vi "Query_ResonantFrequency_Sub_VI.vi"(9 "error in (no error)":errorcluster, 11 "connection ID":refnum<k5>) -> (0 "error out":errorcluster, 2 "connection ID_out":refnum<k5>, 3 "Resonant Frequencies":string)   [LabVIEW 2017]
panel:
  out "data out":string
  out "*(type *) &x 3":u8
  out "substring":string
  out "data out 2":string
  out "x+y":i32
  out "array":string[](array[string])
  out "*(type *) &x":u8
  # "OUTPUT"
  # "INPUT"
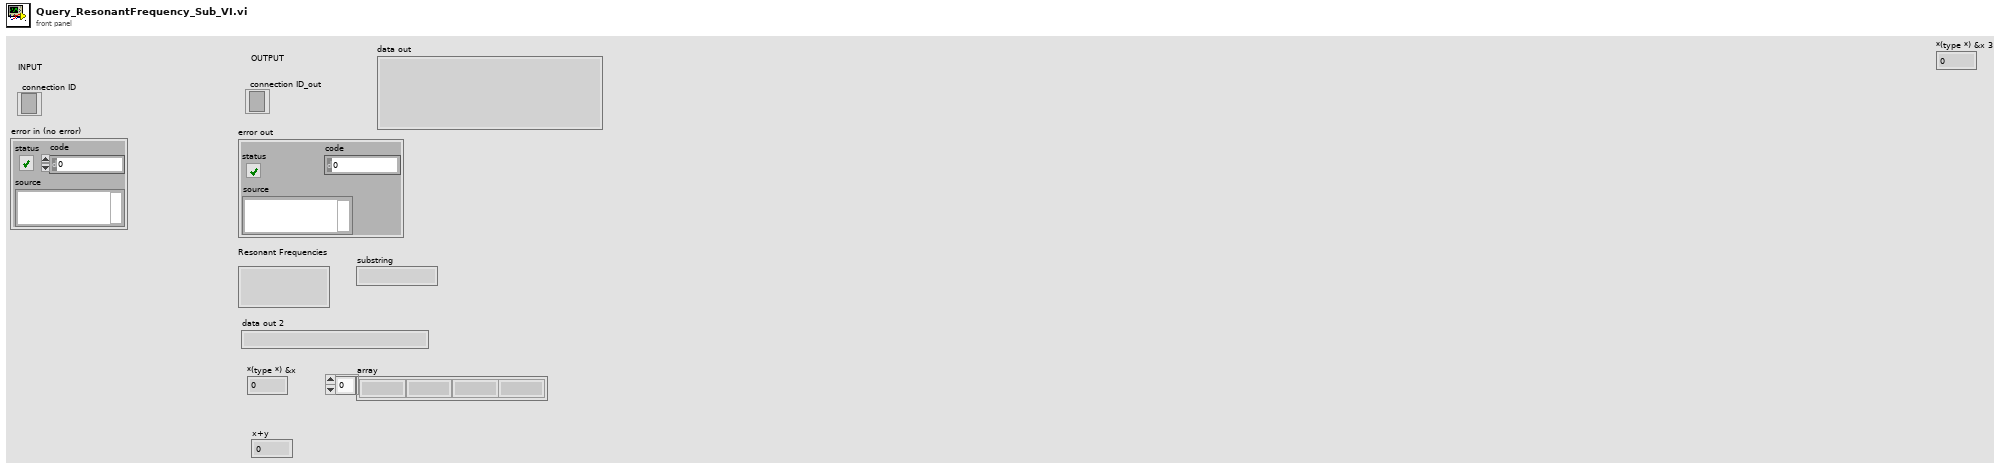
[diagram p1: front panel]
types:
  T1 = enum16{"Standard", "Buffered", "CRLF", "Immediate"}
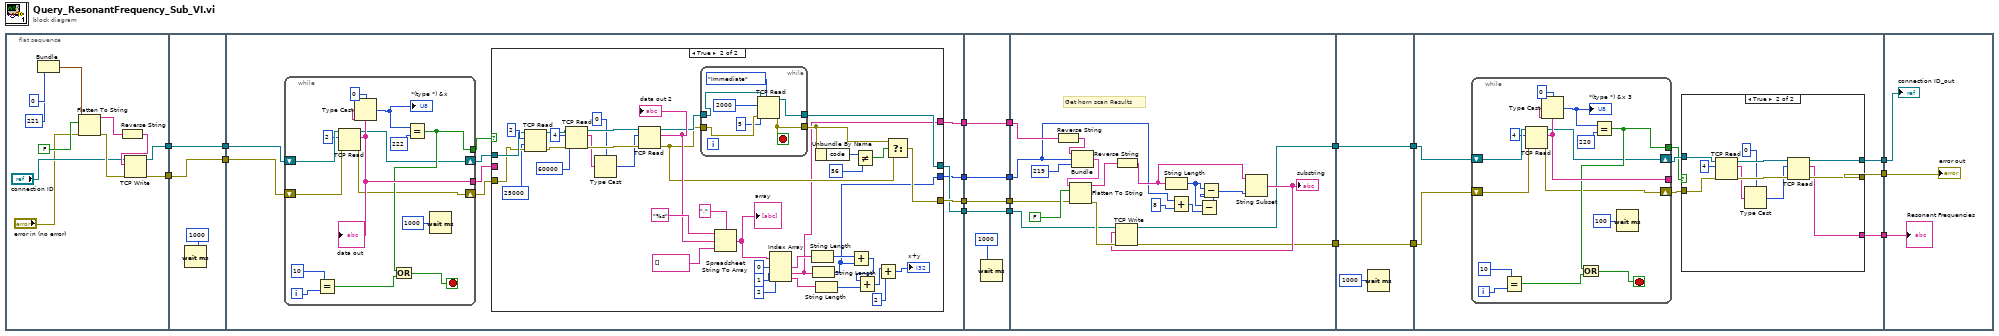
[diagram p0: block diagram]
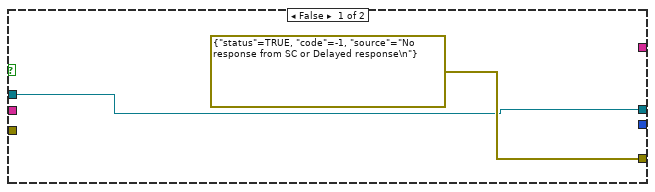
[diagram p2: hidden frame]
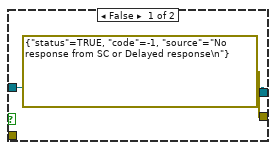
[diagram p3: hidden frame]
diagram:
  n1 = flat-sequence {
    tunnel: [w26] -> w19
    tunnel: [w25] -> w16
    tunnel: w19 -> [w32]
    tunnel: [w32] -> w18
    tunnel: [w31] -> w17
    tunnel: w16 -> [w31]
    tunnel: w18 -> [w41]
    tunnel: w17 -> [w40]
    tunnel: [w38] -> w14
    tunnel: [w36] -> w12
    tunnel: [w35] -> w11
    tunnel: [w34] -> w8
    tunnel: [w110] -> w15
    tunnel: w14 -> [w110]
    tunnel: [w109] -> w13
    tunnel: w12 -> [w109]
    tunnel: w11 -> [w108]
    tunnel: [w108] -> w10
    tunnel: [w107] -> w9
    tunnel: w8 -> [w107]
    tunnel: w15 -> [w127]
    tunnel: w13 -> [w126]
    tunnel: w10 -> [w119]
    tunnel: w9 -> [w124]
    tunnel: [w116] -> w6
    tunnel: [w115] -> w4
    tunnel: [w133] -> w7
    tunnel: w6 -> [w133]
    tunnel: [w132] -> w5
    tunnel: w4 -> [w132]
    tunnel: w7 -> [w141]
    tunnel: w5 -> [w140]
    tunnel: [w138] -> w3
    tunnel: [w137] -> w2
    tunnel: [w136] -> w1
    tunnel: w3 -> [w171]
    tunnel: w2 -> [w170]
    tunnel: w1 -> [w172]
    frame #0 {
      n2 = Bundle(0, 221) -> (w24:cluster{i32, i32})  [unwired: 1 in]
      n3 = Flatten To String(anything=w24, prepend array or string size? (T)=FALSE, error in (no error)="error in (no error)") -> (data string=w23:string, error out=w29:errorcluster)  [unwired: 1 in, 1 out]
      n4 = Reverse String(1:w23) -> (0:w22:string)
      n5 = TCP Write(connection ID="connection ID", data in=w22, error in (no error)=w29) -> (connection ID out=w26:refnum<k5>, error out=w25:errorcluster)  [unwired: 1 in, 1 out]
    }
    frame #1 {
      n6 = Wait (ms)(milliseconds to wait=u32 1000) -> ()  [unwired: 1 out]
    }
    frame #2 {
      n7 = while {
        shift-right: [w47] -> w37
        shift-left: w41 -> [w49]
        shift-right: [w46] -> w39
        shift-left: w40 -> [w48]
        tunnel: [w51] -> w43
        tunnel: [w55] -> w42
        i -> [w54]
        stop <- w52 stop-if-true
        n8 = Equal?(x=10, y=w54) -> (x = y?=w50:bool)
        n9 = TCP Read(connection ID=w49, bytes to read=2, error in (no error)=w48) -> (connection ID out=w47:refnum<k5>, data out=w55:string, error out=w46:errorcluster)  [unwired: 2 in]
        "data out" <- w55
        n10 = Type Cast(type=u8 0, x=w55) -> (*(type *) &x=w57:u8)
        "*(type *) &x" <- w57
        n11 = Equal?(x=w57, y=u8 222) -> (x = y?=w51:bool)
        n12 = Or(x=w51, y=w50) -> (x .or. y?=w52:bool)
        n13 = Wait (ms)(milliseconds to wait=u32 1000) -> ()  [unwired: 1 out]
      }
      n14 = case shown="True" w43 {
        tunnel: w42 -> [_ _]
        tunnel: w39 -> [_ w63]
        tunnel: [errorcluster {"status"=TRUE, "code"=-1, "source"="No response from SC or Delayed response\n"} ("error constant") w69] -> w38
        tunnel: w37 -> [w59 w65]
        tunnel: [w59 w75] -> w36
        tunnel: [_ w67] -> w35
        tunnel: [_ w68] -> w34
        frame False {
        }
        frame True {
          n15 = TCP Read(connection ID=w65, bytes to read=2, error in (no error)=w63, 9:25000 ("timeout ms (25000)")) -> (connection ID out=w64:refnum<k5>, error out=w62:errorcluster)  [unwired: 1 in, 1 out]
          n16 = TCP Read(connection ID=w64, bytes to read=4, error in (no error)=w62, 9:60000 ("timeout ms (25000)")) -> (connection ID out=w82:refnum<k5>, data out=w81:string, error out=w83:errorcluster)  [unwired: 1 in]
          n17 = Type Cast(type=u8 0, x=w81) -> (*(type *) &x=w79:u8)
          n18 = TCP Read(connection ID=w82, bytes to read=w79, error in (no error)=w83) -> (connection ID out=w76:refnum<k5>, data out=w78:string, error out=w70:errorcluster)  [unwired: 2 in]
          "data out 2" <- w78
          n19 = while {
            tunnel: w70 -> [w105]
            tunnel: w76 -> [w106]
            tunnel: [w104] -> w75
            tunnel: [w100] -> w74
            stop <- w100 stop-if-true
            n20 = TCP Read(connection ID=w106, bytes to read=2000, error in (no error)=w105, 7:T1."Immediate" ("mode (standard)"), 9:5 ("timeout ms (25000)")) -> (connection ID out=w104:refnum<k5>, error out=w100:errorcluster)  [unwired: 1 out]
          }
          n21 = Spreadsheet String To Array(delimiter (Tab)=",", format string="%s", spreadsheet string=w78, array type (2D Dbl)=string[] []) -> (array=w96:string[])
          "array" <- w96
          n22 = Index Array(array=w96, index #1=0 ("index"), index #2=1 ("index"), index #3=2 ("index")) -> (element #1=w85:string, element #2=w68:string, element #3=w92:string)
          n23 = String Length(string=w85) -> (length=w86:i32)
          n24 = String Length(string=w68) -> (length=w67:i32)
          n25 = Unbundle By Name(w74) -> ("code"=w73:i32)
          n26 = String Length(string=w92) -> (length=w90:i32)
          n27 = Add(x=w86, y=w67) -> (x+y=w91:i32)
          n28 = Not Equal?(x=w73, y=56) -> (x != y?=w71:bool)
          n29 = Add(x=w91, y=w90) -> (x+y=w89:i32)
          n30 = Add(x=w89, y=2) -> (x+y=→"x+y":i32)
          n31 = Select(t=w74, s=w71, f=w70) -> (s? t:f=w69:errorcluster)
        }
      }
    }
    frame #3 {
      n32 = Wait (ms)(milliseconds to wait=u32 1000) -> ()  [unwired: 1 out]
    }
    frame #4 {
      # "Get horn scan Results"
      n33 = Reverse String(1:w124) -> (0:w123:string)
      n34 = Bundle(w123, w119, 219) -> (w122:cluster{string, i32, i32})  [unwired: 1 in]
      n35 = Flatten To String(anything=w122, prepend array or string size? (T)=FALSE, error in (no error)=w127) -> (data string=w128:string, error out=w129:errorcluster)  [unwired: 1 in, 1 out]
      n36 = Reverse String(1:w128) -> (0:w121:string)
      n37 = String Length(string=w121) -> (length=w114:i32)
      n38 = Add(x=w119, y=8 ("bytes to read")) -> (x+y=w113:i32)
      n39 = Subtract(x=w114, y=w113) -> (x-y=w118:i32)
      n40 = Subtract(x=w114, y=w118) -> (x-y=w112:i32)
      n41 = String Subset(string=w121, length (rest)=w112) -> (substring=w117:string)  [unwired: 1 in]
      "substring" <- w117
      n42 = TCP Write(connection ID=w126, data in=w117, error in (no error)=w129) -> (connection ID out=w115:refnum<k5>, error out=w116:errorcluster)  [unwired: 1 in, 1 out]
    }
    frame #5 {
      n43 = Wait (ms)(milliseconds to wait=u32 1000) -> ()  [unwired: 1 out]
    }
    frame #6 {
      n44 = while {
        shift-right: [w158] -> w139
        shift-left: w140 -> [w160]
        shift-right: [w157] -> w134
        shift-left: w141 -> [w159]
        tunnel: [w162] -> w135
        tunnel: [w166] -> _
        i -> [w165]
        stop <- w163 stop-if-true
        n45 = Equal?(x=10, y=w165) -> (x = y?=w161:bool)
        n46 = TCP Read(connection ID=w160, bytes to read=4, error in (no error)=w159) -> (connection ID out=w158:refnum<k5>, data out=w166:string, error out=w157:errorcluster)  [unwired: 2 in]
        n47 = Type Cast(type=u8 0, x=w166) -> (*(type *) &x=w168:u8)
        "*(type *) &x 3" <- w168
        n48 = Equal?(x=w168, y=u8 220) -> (x = y?=w162:bool)
        n49 = Or(x=w162, y=w161) -> (x .or. y?=w163:bool)
        n50 = Wait (ms)(milliseconds to wait=u32 100) -> ()  [unwired: 1 out]
      }
      n51 = case shown="True" w135 {
        tunnel: w139 -> [w142 w148]
        tunnel: [w142 w147] -> w138
        tunnel: [errorcluster {"status"=TRUE, "code"=-1, "source"="No response from SC or Delayed response\n"} ("error constant") w146] -> w137
        tunnel: [_ w145] -> w136
        tunnel: w134 -> [_ w144]
        frame False {
        }
        frame True {
          n52 = TCP Read(connection ID=w148, bytes to read=4, error in (no error)=w144) -> (connection ID out=w152:refnum<k5>, data out=w151:string, error out=w153:errorcluster)  [unwired: 2 in]
          n53 = Type Cast(type=u8 0, x=w151) -> (*(type *) &x=w149:u8)
          n54 = TCP Read(connection ID=w152, bytes to read=w149, error in (no error)=w153) -> (connection ID out=w147:refnum<k5>, data out=w145:string, error out=w146:errorcluster)  [unwired: 2 in]
        }
      }
    }
    frame #7 {
      "error out" <- w170
      "Resonant Frequencies" <- w172
      "connection ID_out" <- w171
    }
  }
